vi "3 Sync - Digital Trigger Showing Drift.vi"() -> ()   [LabVIEW 2023]
doc: "This example demonstrates how to acquire a single buffer of voltage measurements using a DAQmx device.\n\nFor instructions on how to connect your signals to the DAQ device, refer to your device documentation."
uses:
  <vilib>/DAQmx/create/channels.llb/DAQmx Create Channel (AI-Voltage-Basic).vi
  <vilib>/DAQmx/configure/timing.llb/DAQmx Timing (Sample Clock).vi
  <vilib>/DAQmx/read.llb/DAQmx Read (Analog Wfm 1Chan NSamp).vi
  <resource>/objmgr/daqmx.rc
  <vilib>/DAQmx/configure/trigger.llb/DAQmx Start Trigger (Digital Edge).vi
  <vilib>/DAQmx/write.llb/DAQmx Write (Digital Bool 1Line 1Point).vi
  <vilib>/DAQmx/configure/timing.llb/DAQmx Timing (Implicit).vi
  <vilib>/DAQmx/create/channels.llb/DAQmx Create Channel (DO-Digital Output).vi
  <vilib>/DAQmx/create/channels.llb/DAQmx Create Channel (CO-Pulse Generation-Frequency).vi
panel:
  in  "stop":bool
  in  "Trigger Output: Line":tag="MIODAQ/port0/line2"
  in  "Device 2: Trigger Input":tag="/cDAQ9189-2628AACMod5/PFI4"
  in  "Device 1: Trigger Input":tag="/MIODAQ/PFI4"
  in  "Square Wave Output: Terminal":tag="/MIODAQ/PFI0"
  in  "Square Wave Output: Source":tag="MIODAQ/ctr0"
  out "Skew":dbl
  in  "Device 2: Analog Input Channel":tag="cDAQ9189-2628AACMod1/ai0"
  out "Waveform Graph":waveform(dbl)[](graph)
  in  "Device 1 & 2: Sample Rate":dbl=100000.0
  in  "Device 1 & 2: Sample Clock Source":tag="OnboardClock"
  in  "Device 1: Analog Input Channel":tag="MIODAQ/ai0"
  # "Channel Settings"
  # "Acquired Data"
  # "Timing Settings"
  # "Trigger Acq Settings"
  # "Output Signal Settings"
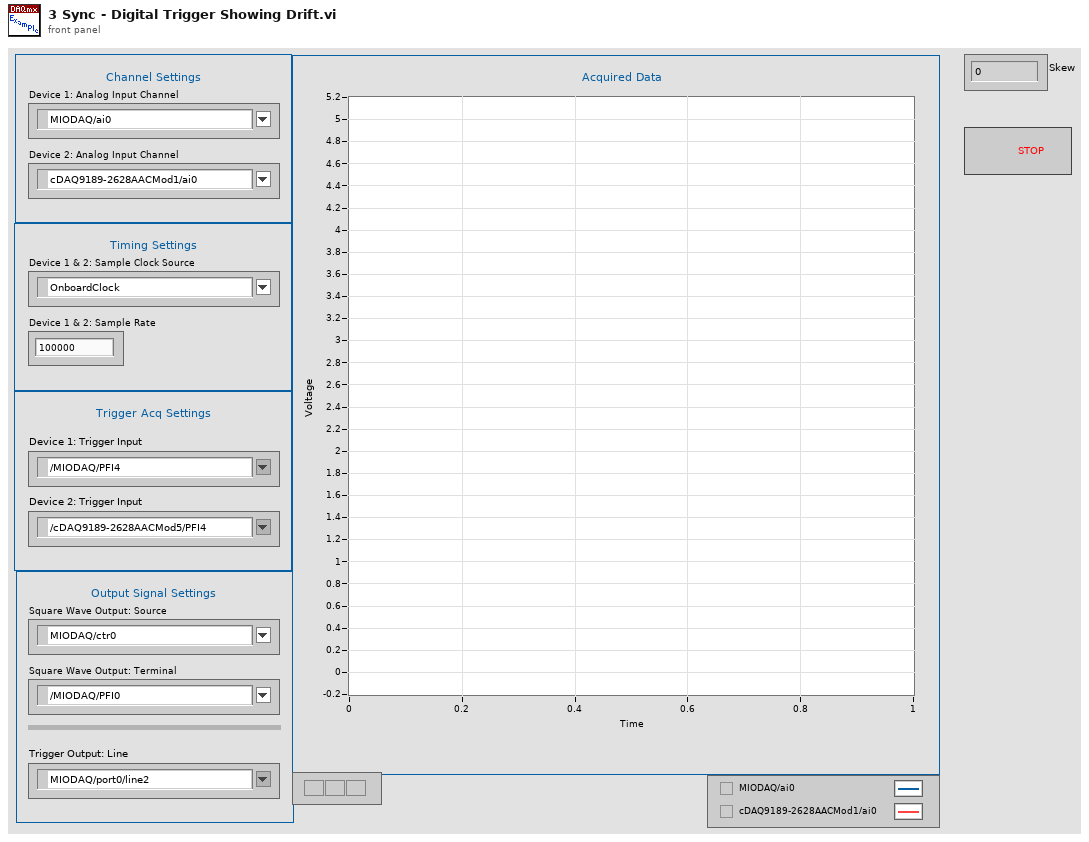
[diagram p1: front panel]
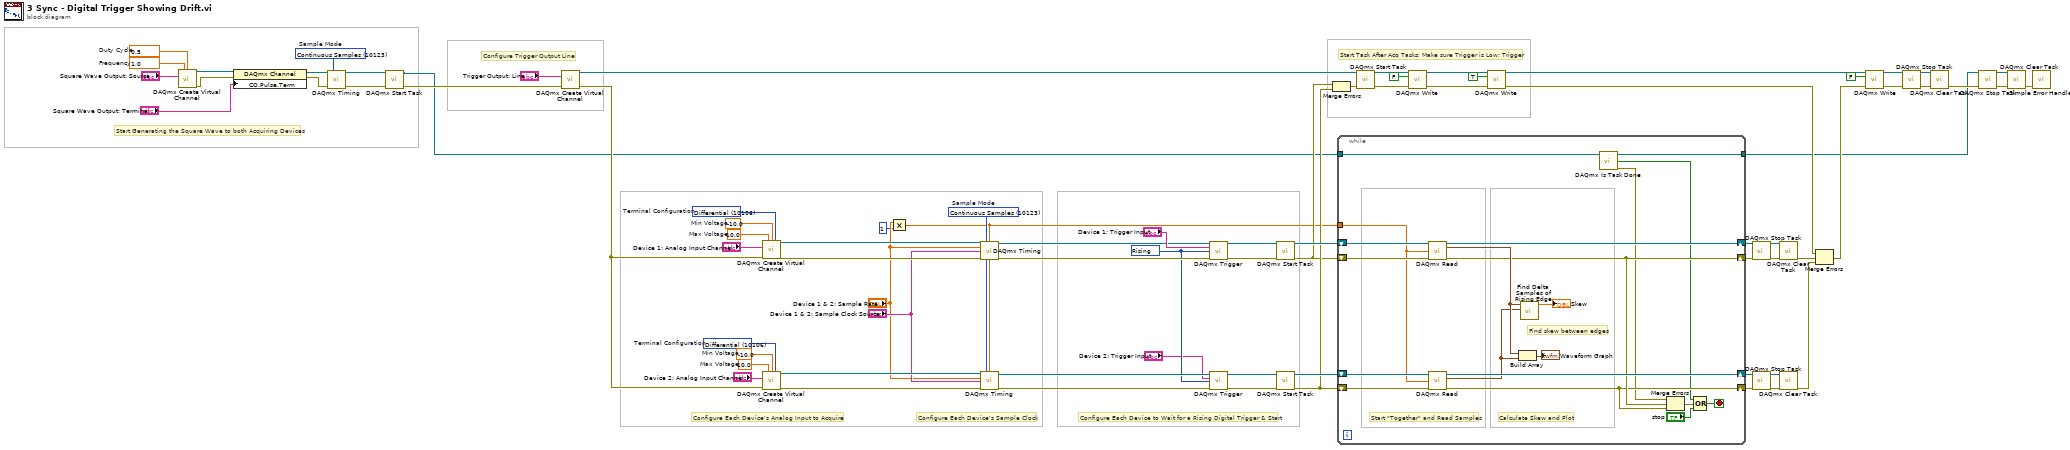
[diagram p0: block diagram]
diagram:
  w28 = 10280 items=["Rising"=10280, "Falling"=10171] ("Digital Start Trigger Edge")
  w53 = 10.0  # Max Voltage
  w52 = -10.0  # Min Voltage
  w51 = 10106 items=["default"=-1, "RSE"=10083, "NRSE"=10078, "Differential"=10106, "Pseudodifferential"=12529]  # Terminal Configuration
  w57 = 10.0  # Max Voltage
  w58 = -10.0  # Min Voltage
  w59 = 10106 items=["default"=-1, "RSE"=10083, "NRSE"=10078, "Differential"=10106, "Pseudodifferential"=12529]  # Terminal Configuration
  w41 = 10123 items=["Finite Samples"=10178, "Continuous Samples"=10123, "Hardware Timed Single Point"=12522]  # Sample Mode
  w75 = 1.0  # Frequency
  w76 = 0.5  # Duty Cycle
  w68 = 10123 items=["Finite Samples"=10178, "Continuous Samples"=10123, "Hardware Timed Single Point"=12522]  # Sample Mode
  # "Start Task After Acq Tasks; Make sure Trigger is Low; Trigger"
  # "Configure Each Device to Wait for a Rising Digital Trigger & Start"
  # "Configure Trigger Output Line"
  # "Configure Each Device's Sample Clock"
  # "Configure Each Device's Analog Input to Acquire"
  # "Start Generating the Square Wave to both Acquiring Devices"
  n1 = call-poly <vilib>:"DAQmx Create Virtual Channel.vi"("frequency"=w75, "duty cycle"=w76, "counter"="Square Wave Output: Source") -> ("task out"=w70:refnum<k21>, "error out"=w71:errorcluster)  [unwired: 11 in]
  n2 = property class="DAQmx Channel"(reference=w70, error in=w71, "CO.Pulse.Term"="Square Wave Output: Terminal") -> (reference out=w74:refnum<k21>, error out=w73:errorcluster)
  n3 = call-poly <vilib>:"DAQmx Timing.vi"("task/channels in"=w74, "sample mode"=w68, "error in"=w73) -> ("task out"=w78:refnum<k21>, "error out"=w77:errorcluster)  [unwired: 11 in]
  n4 = call <vilib>:"DAQmx Start Task.vi"("task/channels in"=w78, "error in"=w77) -> ("task out"=w2:refnum<k21>, "error out"=w64:errorcluster)  [unwired: 12 in]
  n5 = call-poly <vilib>:"DAQmx Create Virtual Channel.vi"("lines"="Trigger Output: Line", "error in"=w64) -> ("task out"=w18:refnum<k21>, "error out"=w25:errorcluster)  [unwired: 12 in]
  n6 = call-poly <vilib>:"DAQmx Create Virtual Channel.vi"("maximum value"=w57, "minimum value"=w58, "input terminal configuration"=w59, "physical channels"="Device 1: Analog Input Channel", "error in"=w25) -> ("task out"=w62:refnum<k21>, "error out"=w63:errorcluster)  [unwired: 9 in]
  n7 = call-poly <vilib>:"DAQmx Create Virtual Channel.vi"("maximum value"=w53, "minimum value"=w52, "input terminal configuration"=w51, "physical channels"="Device 2: Analog Input Channel", "error in"=w25) -> ("task out"=w50:refnum<k21>, "error out"=w49:errorcluster)  [unwired: 9 in]
  n8 = Multiply(x="Device 1 & 2: Sample Rate", y=1) -> (x*y=w4:dbl)
  n9 = call-poly <vilib>:"DAQmx Timing.vi"("task/channels in"=w62, "sample mode"=w41, "samples per channel"=w4, "rate"="Device 1 & 2: Sample Rate", "source"="Device 1 & 2: Sample Clock Source", "error in"=w63) -> ("task out"=w34:refnum<k21>, "error out"=w33:errorcluster)  [unwired: 8 in]
  n10 = call-poly <vilib>:"DAQmx Timing.vi"("task/channels in"=w50, "sample mode"=w41, "samples per channel"=w4, "rate"="Device 1 & 2: Sample Rate", "source"="Device 1 & 2: Sample Clock Source", "error in"=w49) -> ("task out"=w31:refnum<k21>, "error out"=w29:errorcluster)  [unwired: 8 in]
  n11 = call-poly <vilib>:"DAQmx Trigger.vi"("task/channels in"=w34, "source"="Device 1: Trigger Input", "edge"=w28, "error in"=w33) -> ("task out"=w32:refnum<k21>, "error out"=w16:errorcluster)  [unwired: 10 in]
  n12 = call-poly <vilib>:"DAQmx Trigger.vi"("task/channels in"=w31, "source"="Device 2: Trigger Input", "edge"=w28, "error in"=w29) -> ("task out"=w30:refnum<k21>, "error out"=w17:errorcluster)  [unwired: 10 in]
  n13 = call <vilib>:"DAQmx Start Task.vi"("task/channels in"=w32, "error in"=w16) -> ("task out"=w61:refnum<k21>, "error out"=w14:errorcluster)  [unwired: 12 in]
  n14 = call <vilib>:"DAQmx Start Task.vi"("task/channels in"=w30, "error in"=w17) -> ("task out"=w42:refnum<k21>, "error out"=w15:errorcluster)  [unwired: 12 in]
  n15 = Merge Errors(w14, w15) -> (w13:errorcluster)
  n16 = while {
    shift-right: [w96] -> w54
    shift-left: w61 -> [w97]
    shift-right: [w95] -> w45
    shift-left: w42 -> [w94]
    shift-right: [w86] -> w46
    shift-left: w15 -> [w90]
    shift-right: [w87] -> w38
    shift-left: w14 -> [w89]
    tunnel: w4 -> [w88]
    tunnel: w2 -> [w82]
    tunnel: [w79] -> w1
    stop <- w83 stop-if-true
    # "Calculate Skew and Plot"
    # "Start \"Together\" and Read Samples"
    # "Find skew between edges"
    n17 = call-poly <vilib>:"DAQmx Read.vi"("task/channels in"=w97, "number of samples per channel"=w88, "error in"=w89) -> ("task out"=w96:refnum<k21>, "data"=w92:waveform(dbl), "error out"=w87:errorcluster)  [unwired: 10 in]
    n18 = call-poly <vilib>:"DAQmx Read.vi"("task/channels in"=w94, "number of samples per channel"=w88, "error in"=w90) -> ("task out"=w95:refnum<k21>, "data"=w91:waveform(dbl), "error out"=w86:errorcluster)  [unwired: 10 in]
    n19 = Build Array(w92, w91) -> (→"Waveform Graph":waveform(dbl)[])
    n20 = call "Find Delta Samples of Rising Edge.vi"("Channel 2"=w91, "Channel 1"=w92) -> ("Sample Offset"=→"Skew":dbl)  [unwired: 9 in]
    n21 = call <vilib>:"DAQmx Is Task Done.vi"("task/channels in"=w82) -> ("task out"=w79:refnum<k21>, "task done?"=w80:bool, "error out"=w81:errorcluster)  [unwired: 12 in]
    n22 = Merge Errors(w81, w87, w86) -> (w85:errorcluster)
    n23 = Compound Arithmetic op=OR(w80, w85, "stop") -> (w83:bool)
  }
  n24 = call <vilib>:"DAQmx Start Task.vi"("task/channels in"=w18, "error in"=w13) -> ("task out"=w24:refnum<k21>, "error out"=w23:errorcluster)  [unwired: 12 in]
  n25 = call-poly <vilib>:"DAQmx Write.vi"("task/channels in"=w24, "data"=FALSE, "error in"=w23) -> ("task out"=w20:refnum<k21>, "error out"=w19:errorcluster)  [unwired: 10 in, 1 out]
  n26 = call-poly <vilib>:"DAQmx Write.vi"("task/channels in"=w20, "data"=TRUE, "error in"=w19) -> ("task out"=w6:refnum<k21>, "error out"=w12:errorcluster)  [unwired: 10 in, 1 out]
  n27 = call <vilib>:"DAQmx Stop Task.vi"("task/channels in"=w54, "error in"=w38) -> ("task out"=w56:refnum<k21>, "error out"=w55:errorcluster)  [unwired: 12 in]
  n28 = call <vilib>:"DAQmx Stop Task.vi"("task/channels in"=w45, "error in"=w46) -> ("task out"=w43:refnum<k21>, "error out"=w44:errorcluster)  [unwired: 12 in]
  n29 = call <vilib>:"DAQmx Clear Task.vi"("task in"=w56, "error in"=w55) -> ("error out"=w39:errorcluster)  [unwired: 13 in]
  n30 = call <vilib>:"DAQmx Clear Task.vi"("task in"=w43, "error in"=w44) -> ("error out"=w40:errorcluster)  [unwired: 13 in]
  n31 = Merge Errors(w12, w39, w40) -> (w5:errorcluster)
  n32 = call-poly <vilib>:"DAQmx Write.vi"("task/channels in"=w6, "data"=FALSE, "error in"=w5) -> ("task out"=w7:refnum<k21>, "error out"=w8:errorcluster)  [unwired: 10 in, 1 out]
  n33 = call <vilib>:"DAQmx Stop Task.vi"("task/channels in"=w7, "error in"=w8) -> ("task out"=w11:refnum<k21>, "error out"=w10:errorcluster)  [unwired: 12 in]
  n34 = call <vilib>:"DAQmx Clear Task.vi"("task in"=w11, "error in"=w10) -> ("error out"=w3:errorcluster)  [unwired: 13 in]
  n35 = call <vilib>:"DAQmx Stop Task.vi"("task/channels in"=w1, "error in"=w3) -> ("task out"=w66:refnum<k21>, "error out"=w67:errorcluster)  [unwired: 12 in]
  n36 = call <vilib>:"DAQmx Clear Task.vi"("task in"=w66, "error in"=w67) -> ("error out"=w65:errorcluster)  [unwired: 13 in]
  n37 = call <vilib>:"Simple Error Handler.vi"("error in (no error)"=w65) -> ()  [unwired: 4 in, 5 out]
